vi "Translation2d_NearestTo.vi"(9 "Other Translations":T1[](array[typedef]) {"Y" format="%14.3f"; "X" format="%14.3f"}, 11 "In Translation":T1 {"Y" format="%14.3f"; "X" format="%14.3f"}) -> (1 "Found":bool, 3 "Nearest Translation":T1 {"Y" format="%14.3f"; "X" format="%14.3f"})   [LabVIEW 2019, in "Trajectory_Library.lvlib"]
doc: "Returns the inverse of the current translation. This is equivalent to rotating by 180 degrees, flipping the point over both axes, or simply negating both components of the translation.\n \nParameters:\n - In Translation - This translation data structure\n\nResult:\n - Out Translation - The inverse of the current translation."
uses:
  Trajectory_Library.lvlib
  TypeDef/TRANSLATION2D.ctl
  Util_CalcDist.vi
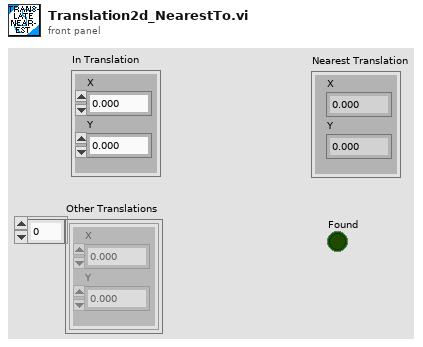
[diagram p1: front panel]
types:
  T1 = typedef "Trajectory_Library.lvlib/TRANSLATION2D.ctl" = cluster{"X":dbl, "Y":dbl}
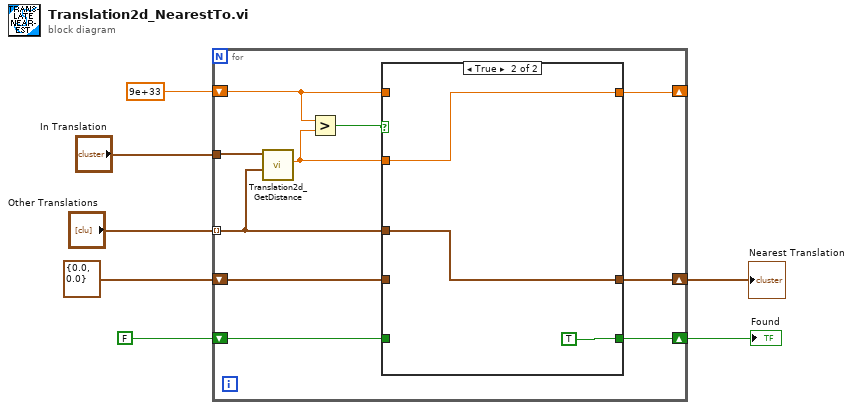
[diagram p0: block diagram]
diagram:
  n1 = for {
    shift-right: [w14] -> _
    shift-left: 9e+33 -> [w10]
    tunnel: "In Translation" -> [w17]
    tunnel: "Other Translations" -> [w15] mode=indexing
    shift-right: [w11] -> w2
    shift-left: FALSE -> [w8]
    shift-right: [w12] -> w1
    shift-left: T1 {"X"=0.0, "Y"=0.0} ("Other Translation") -> [w9]
    n2 = call "Translation2d_GetDistance.vi"("other Translation"=w15, "In Translation"=w17) -> ("Distance"=w13:dbl)  [unwired: 9 in]
    n3 = Greater?(x=w10, y=w13) -> (0:w16:bool)
    n4 = case shown="True" w16 {
      tunnel: w15 -> [_ w22]
      tunnel: [w20 w23] -> w14
      tunnel: w13 -> [_ w23]
      tunnel: [w19 w22] -> w12
      tunnel: [w18 TRUE] -> w11
      tunnel: w10 -> [w20 _]
      tunnel: w9 -> [w19 _]
      tunnel: w8 -> [w18 _]
      frame False {
      }
      frame True {
      }
    }
  }
  "Nearest Translation" <- w1
  "Found" <- w2
